vi "AuMT8852B Modulation Index Results Query.vi"(8 "error in (no error)":errorcluster, 11 "VISA session":refnum<visa-resource-name>) -> (0 "error out":errorcluster, 2 "error code":i32, 3 "VISA session out":refnum<visa-resource-name>, 4 "Results":T1 {"Delta f2 avg / delta f1 avg" format="%.2f"; "Delta f2 average (kHz)" format="%.2f"; "Delta f2 maximum (kHz)" format="%.2f"; "Delta f1 average (kHz)" format="%.2f"; "Delta f1 maximum (kHz)" format="%.2f"})   [LabVIEW 2017]
doc: "Anritsu MT8852B Bluetooth Tester\n\nReturns the results of the Modulation Characteristics test.\n\nOUTPUTS\nResults - measurements made during the test."
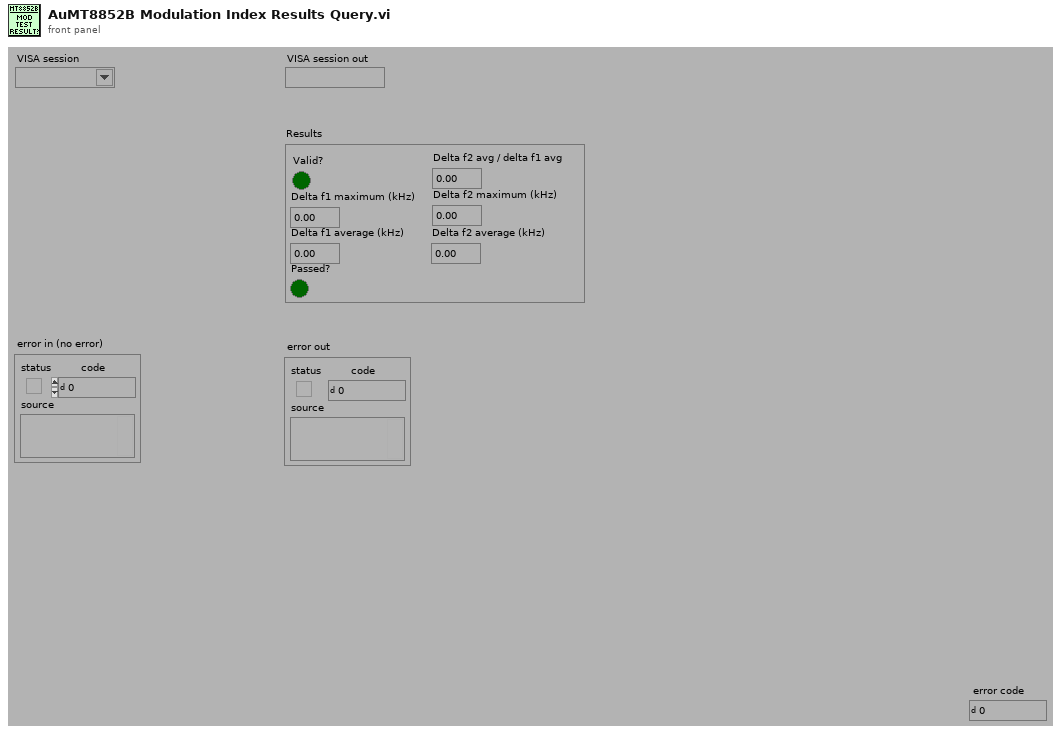
[diagram p1: front panel]
types:
  T1 = cluster{"Delta f1 maximum (kHz)":dbl, "Delta f1 average (kHz)":dbl, "Delta f2 maximum (kHz)":dbl, "Delta f2 average (kHz)":dbl, "Passed?":bool, "Delta f2 avg / delta f1 avg":dbl, "Valid?":bool}
  T2 = enum16{"Simulate", "Range check", "Cache", "Query instrument status"}
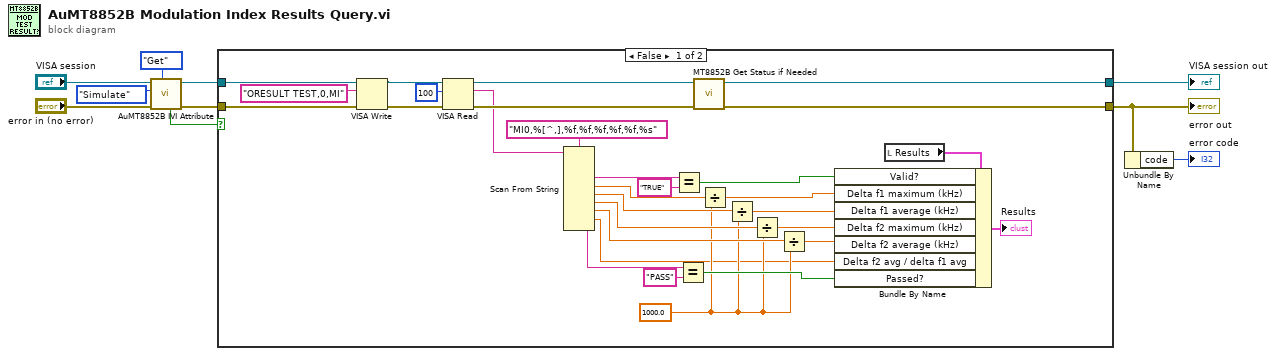
[diagram p0: block diagram]
diagram:
  n1 = call <instrlib>:"AuMT8852B IVI Attribute.vi"("Set/Get (Set)"=enum16{"Set", "Get"}."Get", "error in (no error)"="error in (no error)", "Flag (Simulate)"=T2."Simulate", "VISA session"="VISA session") -> ("error out"=w7:errorcluster, "VISA session out"=w9:refnum<visa-resource-name>, "Value out"=w3:bool)  [unwired: 5 in]
  n2 = case shown="False" w3 {
    tunnel: [w27 w42] -> w10
    tunnel: [w26 w41] -> w1
    tunnel: w9 -> [w39 w42]
    tunnel: w7 -> [w38 w41]
    frame False {
      w12 = 1000.0 ("y")
      n3 = VISA Write(VISA resource name=w39, write buffer="ORESULT TEST,0,MI" ("write buffer (\"\")"), error in (no error)=w38) -> (VISA resource name out=w37:refnum<visa-resource-name>, error out=w36:errorcluster)  [unwired: 1 out]
      n4 = VISA Read(VISA resource name=w37, byte count=u32 100 ("byte count (0)"), error in (no error)=w36) -> (VISA resource name out=w23:refnum<visa-resource-name>, read buffer=w21:string, error out=w22:errorcluster)  [unwired: 1 out]
      n5 = Scan From String(format string="MI0,%[^,],%f,%f,%f,%f,%f,%s" ("Format String"), input string=w21) -> (output 1=w31:string, output 2=w13:dbl, output 3=w16:dbl, output 4=w17:dbl, output 5=w19:dbl, output 6=w11:dbl, output 7=w25:string)  [unwired: 9 in, 3 out]
      n6 = Equal?(x=w31, y="TRUE") -> (x = y?=w32:bool)
      n7 = Equal?(x=w25, y="PASS") -> (x = y?=w24:bool)
      n8 = call <instrlib>:"MT8852B Get Status if Needed.vi"("error in (no error)"=w22, "VISA session"=w23) -> ("error out"=w26:errorcluster, "VISA session out"=w27:refnum<visa-resource-name>)  [unwired: 8 in]
      n9 = Divide(x=w13, y=w12) -> (x/y=w14:dbl)
      n10 = Divide(x=w16, y=w12) -> (x/y=w15:dbl)
      n11 = Divide(x=w17, y=w12) -> (x/y=w18:dbl)
      n12 = Divide(x=w19, y=w12) -> (x/y=w20:dbl)
      n13 = local read "Results"() -> (w33:T1)
      n14 = Bundle By Name(cluster=w33, "Valid?"=w32, "Delta f1 maximum (kHz)"=w14, "Delta f1 average (kHz)"=w15, "Delta f2 maximum (kHz)"=w18, "Delta f2 average (kHz)"=w20, "Delta f2 avg / delta f1 avg"=w11, "Passed?"=w24) -> (→"Results":T1)
    }
    frame True {
    }
  }
  "error out" <- w1
  "VISA session out" <- w10
  n15 = Unbundle By Name(w1) -> ("code"=→"error code":i32)
